vi "PathPlanner_CommandUtil_TypeFromString.vi"(11 "Type string":string) -> (3 "Type":T1)   [LabVIEW 2019, in "PathPlanner24.lvlib"]
doc: "Get the command utility type enum from a string\n\nInputs:\n -- Type string - string - string to evaluate for command util type\n\nOutputs:\n -- type - enum - Evaluated command util type."
uses:
  PathPlanner24.lvlib
  ENum/PathPlanner_CommandUtilType_ENUM.ctl
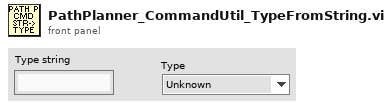
[diagram p1: front panel]
types:
  T1 = typedef "PathPlanner24.lvlib/PathPlanner_CommandUtilType_ENUM.ctl" = enum16{"Unknown", "Wait", "Named", "Path", "Sequential", "Parallel", "Race", "Deadline"}
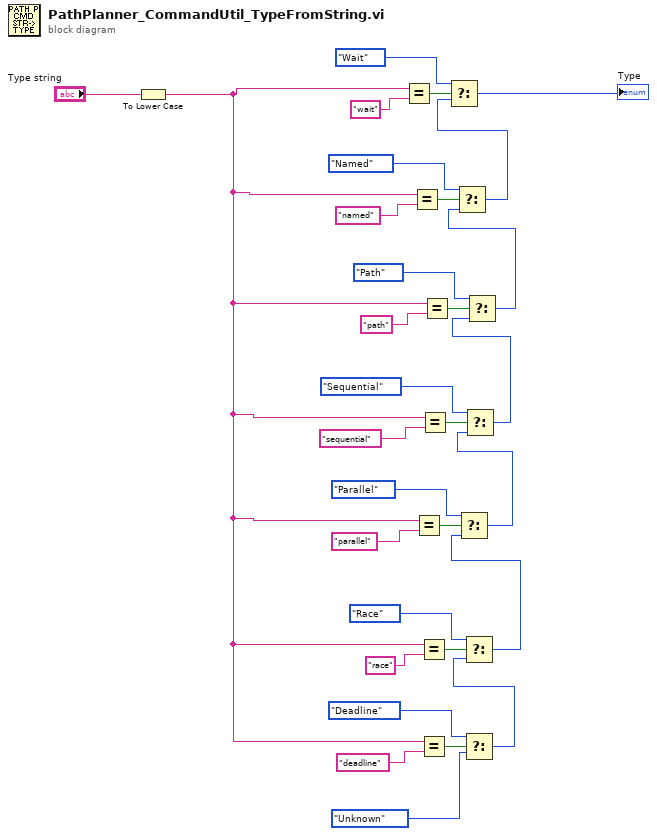
[diagram p0: block diagram]
diagram:
  n1 = To Lower Case(string="Type string") -> (all lower case string=w8:string)
  n2 = Equal?(x=w8, y="wait") -> (x = y?=w30:bool)
  n3 = Equal?(x=w8, y="named") -> (x = y?=w27:bool)
  n4 = Equal?(x=w8, y="parallel") -> (x = y?=w18:bool)
  n5 = Equal?(x=w8, y="race") -> (x = y?=w15:bool)
  n6 = Equal?(x=w8, y="deadline") -> (x = y?=w12:bool)
  n7 = Equal?(x=w8, y="sequential") -> (x = y?=w21:bool)
  n8 = Equal?(x=w8, y="path") -> (x = y?=w24:bool)
  n9 = Select(t=PathPlanner_CommandUtilType_ENUM."Deadline" ("Type"), s=w12, f=PathPlanner_CommandUtilType_ENUM."Unknown" ("Type")) -> (s? t:f=w7:T1)
  n10 = Select(t=PathPlanner_CommandUtilType_ENUM."Race" ("Type"), s=w15, f=w7) -> (s? t:f=w6:T1)
  n11 = Select(t=PathPlanner_CommandUtilType_ENUM."Parallel" ("Type"), s=w18, f=w6) -> (s? t:f=w5:T1)
  n12 = Select(t=PathPlanner_CommandUtilType_ENUM."Sequential" ("Type"), s=w21, f=w5) -> (s? t:f=w4:T1)
  n13 = Select(t=PathPlanner_CommandUtilType_ENUM."Path" ("Type"), s=w24, f=w4) -> (s? t:f=w3:T1)
  n14 = Select(t=PathPlanner_CommandUtilType_ENUM."Named" ("Type"), s=w27, f=w3) -> (s? t:f=w2:T1)
  n15 = Select(t=PathPlanner_CommandUtilType_ENUM."Wait" ("Type"), s=w30, f=w2) -> (s? t:f=→"Type":T1)
